vi "GetTerms4.vi"(0 "XRef":T11, 1 "State In":T10) -> (14 "Terms":T2, 15 "Fatal Error Out":T1)   [LabVIEW 2015, in "LVJSON.lvlib" / "Build JSON Array.xnode"]
uses:
  Build JSON Array.xnode
  <vilib>/XNodeSupport/XNodeXNodeRef.ctl
  State.ctl
  <vilib>/XNodeSupport/XNodeTerm4Array.ctl
  <vilib>/XNodeSupport/XNodeTerm4.ctl
  <vilib>/XNodeSupport/XNodeString.ctl
  <vilib>/XNodeSupport/XNodeVariant.ctl
  <vilib>/XNodeSupport/XNodeRect32.ctl
  <vilib>/XNodeSupport/XNodeInt.ctl
  <vilib>/XNodeSupport/XNodeBool.ctl
  <vilib>/XNodeSupport/XNodeTermDirection.ctl
  <vilib>/XNodeSupport/XNodeErrorCluster.ctl
  JSON Datatype/JSON Null.lvclass
  dimensions.vi
  <vilib>/XNodeSupport/NI_XNodeSupport.lvlib
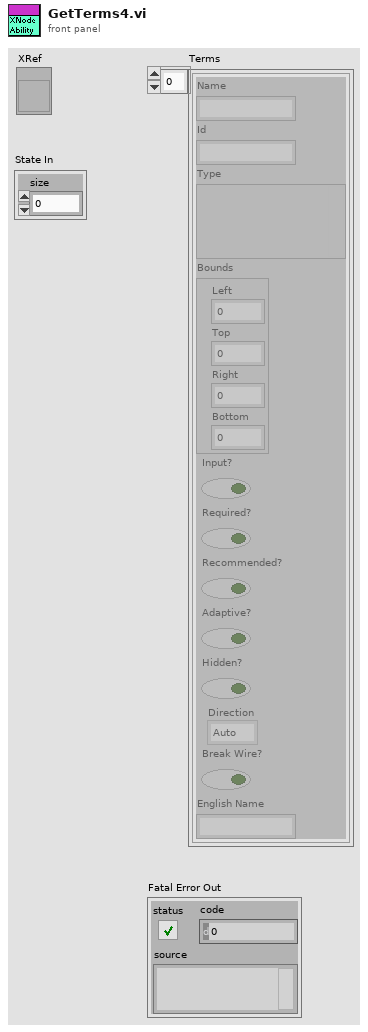
[diagram p1: front panel]
types:
  T1 = typedef "NI_XNodeSupport.lvlib/XNodeErrorCluster.ctl" = errorcluster
  T2 = typedef "NI_XNodeSupport.lvlib/XNodeTerm4Array.ctl" = T3[]
  T3 = typedef "NI_XNodeSupport.lvlib/XNodeTerm4.ctl" = cluster{"Name":T4, "Id":T4, "Type":T5, "Bounds":T6, "Input?":T8, "Required?":T8, "Recommended?":T8, "Adaptive?":T8, "Hidden?":T8, "Direction":T9, "Break Wire?":T8, "English Name":T4}
  T4 = typedef "NI_XNodeSupport.lvlib/XNodeString.ctl" = string
  T5 = typedef "NI_XNodeSupport.lvlib/XNodeVariant.ctl" = variant
  T6 = typedef "NI_XNodeSupport.lvlib/XNodeRect32.ctl" = cluster{"Left":T7, "Top":T7, "Right":T7, "Bottom":T7}
  T7 = typedef "NI_XNodeSupport.lvlib/XNodeInt.ctl" = i32
  T8 = typedef "NI_XNodeSupport.lvlib/XNodeBool.ctl" = bool
  T9 = typedef "NI_XNodeSupport.lvlib/XNodeTermDirection.ctl" = enum32{"Auto", "Up", "Down", "Left", "Right", "Center"}
  T10 = typedef "LVJSON.lvlib/Build JSON Array.xnode/State.ctl" = cluster{"size":u32}
  T11 = typedef "NI_XNodeSupport.lvlib/XNodeXNodeRef.ctl" = refnum<vi>
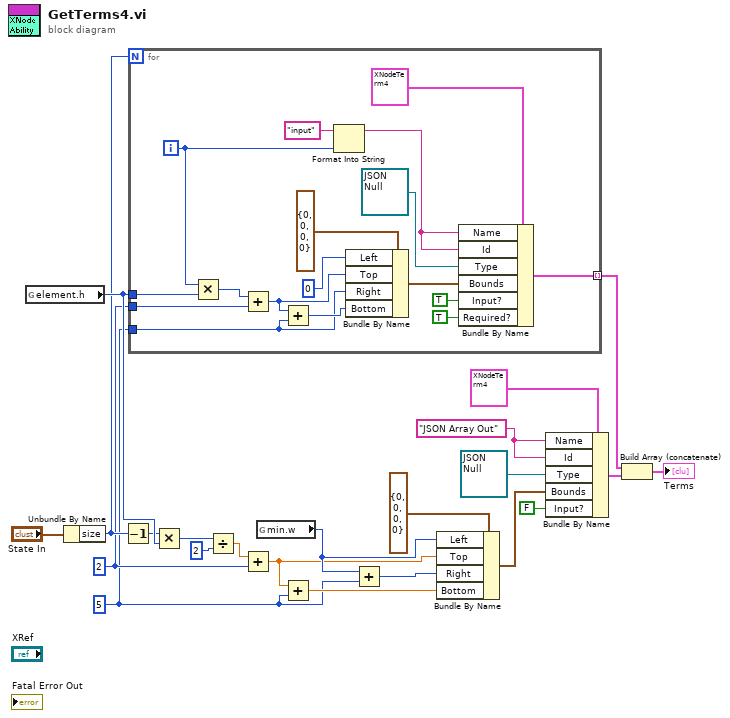
[diagram p0: block diagram]
diagram:
  w2 = 2 ("y")
  w10 = T4 "JSON Array Out" ("Name")
  w1 = T7 5 ("Right")
  n1 = global read "dimensions.vi" "element.h"() -> (w9:i16)
  n2 = Unbundle By Name("State In") -> ("size"=w6:u32)
  n3 = Decrement(x=w6) -> (x-1=w5:u32)
  n4 = for {
    N: w6 -> [_]
    tunnel: [w33] -> w13 mode=indexing
    tunnel: w9 -> [w30]
    tunnel: w2 -> [w24]
    tunnel: w1 -> [w23]
    i -> [w25]
    n5 = Multiply(x=w25, y=w30) -> (x*y=w27:i32)
    n6 = Add(x=w27, y=w24) -> (x+y=w26:i32)
    n7 = Add(x=w26, y=w23) -> (x+y=w28:T7)
    n8 = Format Into String(initial string="input", w25) -> (resulting string=w37:string)  [unwired: 2 in, 1 out]
    n9 = Bundle By Name(cluster=T6 {"Left"=0, "Top"=0, "Right"=0, "Bottom"=0} ("Bounds"), "Left"=T7 0, "Top"=w26, "Right"=w23, "Bottom"=w28) -> (w29:T6)
    n10 = Bundle By Name(cluster=T3 {"Name"="", "Id"="", "Type"=variant, "Bounds"={"Left"=0, "Top"=0, "Right"=0, "Bottom"=0}, "Input?"=FALSE, "Required?"=FALSE, "Recommended?"=FALSE, "Adaptive?"=FALSE, "Hidden?"=FALSE, "Direction"=enum."Auto", "Break Wire?"=FALSE, "English Name"=""} ("Term 4"), "Name"=w37, "Id"=w37, "Type"=refnum<class "JSON Null.lvclass"> refnum ("LVJSON.lvlib:JSON Null.lvclass"), "Bounds"=w29, "Input?"=T8 TRUE, "Required?"=T8 TRUE) -> (w33:T3)
  }
  n11 = Multiply(x=w5, y=w9) -> (x*y=w8:u32)
  n12 = Divide(x=w8, y=u32 2) -> (x/y=w4:dbl)
  n13 = Add(x=w4, y=w2) -> (x+y=w3:dbl)
  n14 = global read "dimensions.vi" "min.w"() -> (w15:i32)
  n15 = Add(x=w3, y=w1) -> (x+y=w21:dbl)
  n16 = Add(x=w15, y=w1) -> (x+y=w14:T7)
  n17 = Bundle By Name(cluster=T6 {"Left"=0, "Top"=0, "Right"=0, "Bottom"=0} ("Bounds"), "Left"=w15, "Top"=w3, "Right"=w14, "Bottom"=w21) -> (w20:T6)
  n18 = Bundle By Name(cluster=T3 {"Name"="", "Id"="", "Type"=variant, "Bounds"={"Left"=0, "Top"=0, "Right"=0, "Bottom"=0}, "Input?"=FALSE, "Required?"=FALSE, "Recommended?"=FALSE, "Adaptive?"=FALSE, "Hidden?"=FALSE, "Direction"=enum."Auto", "Break Wire?"=FALSE, "English Name"=""} ("Term 4"), "Name"=w10, "Id"=w10, "Type"=refnum<class "JSON Null.lvclass"> refnum ("LVJSON.lvlib:JSON Null.lvclass"), "Bounds"=w20, "Input?"=T8 FALSE) -> (w12:T3)
  n19 = Build Array (concatenate)(w13, w12) -> (→"Terms":T3[])
